vi "open_pneumatics.vi"(8 "error in (no error)":errorcluster) -> (0 "error out":errorcluster)   [LabVIEW 2020]
uses:
  <vilib>/Rock Robotics/WPI/Solenoid/WPI_SolenoidChannel.ctl
  <vilib>/Rock Robotics/WPI/Utilities/WPI_GetSetVariantRefNum.vi
  <vilib>/Rock Robotics/WPI/Solenoid/WPI_SolenoidOpenDouble.vi
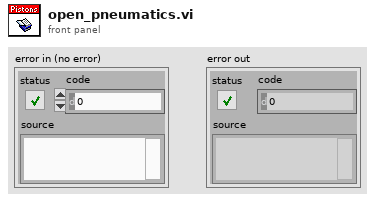
[diagram p1: front panel]
types:
  T1 = typedef "WPI_CompressorDevRef.ctl" = cluster{"DevStatus":errorcluster, "Pneumatics Control Module":u8}
  T2 = typedef "WPI_SolenoidChannel.ctl" = enum8{"Solenoid 0", "Solenoid 1", "Solenoid 2", "Solenoid 3", "Solenoid 4", "Solenoid 5", "Solenoid 6", "Solenoid 7", "Solenoid 8", "Solenoid 9", "Solenoid 10", "Solenoid 11", "Solenoid 12", "Solenoid 13", "Solenoid 14", "Solenoid 15", "Invalid"}
  T3 = typedef "WPI_SolenoidDevRef.ctl" = cluster{"DevStatus":errorcluster, "Pneumatics Control Module":u8, "Forward Solenoid Channel":T2, "Reverse Solenoid Channel":T2}
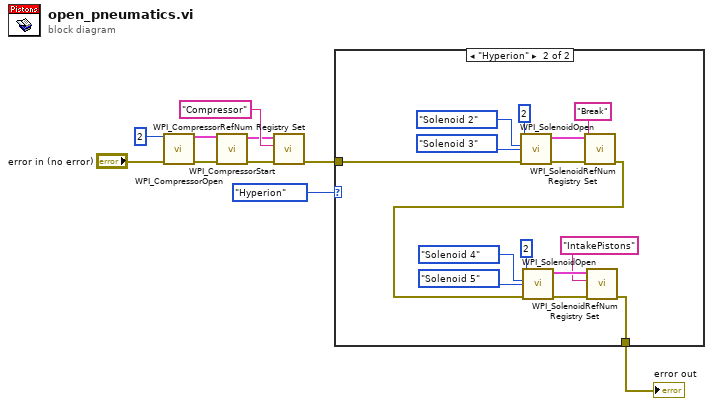
[diagram p0: block diagram]
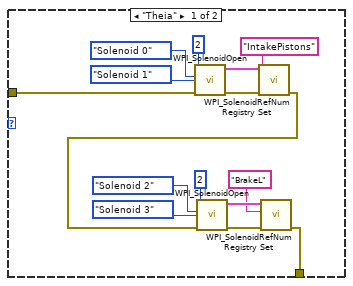
[diagram p2: hidden frame]
diagram:
  n1 = call <vilib>:"WPI_CompressorOpen.vi"("Pneumatics device (def)"=u8 2, "error in (no error)"="error in (no error)") -> ("CompressorDevRef"=w5:T1, "error out"=w6:errorcluster)  [unwired: 12 in]
  n2 = call <vilib>:"WPI_CompressorStart.vi"("error in (no error)"=w6, "CompressorDevRef"=w5) -> ("error out"=w3:errorcluster, "CompressorDevRef"=w4:T1)  [unwired: 8 in]
  n3 = call <vilib>:"WPI_CompressorRefNum Registry Set.vi"("error in (no error)"=w3, "refnum name"="Compressor", "CompressorDevRef"=w4) -> ("error out"=w10:errorcluster)  [unwired: 7 in, 1 out]
  n4 = case shown="\"Hyperion\"" enum16{"Theia", "Hyperion"}."Hyperion" {
    tunnel: w10 -> [w25 w40]
    tunnel: [w11 w26] -> w2
    frame "Theia" {
      n5 = call-poly <vilib>:"WPI_SolenoidOpen.vi"("error in (no error)"=w25, "Reverse Solenoid Channel"=WPI_SolenoidChannel."Solenoid 1", "Forward Solenoid Channel"=WPI_SolenoidChannel."Solenoid 0", "Pneumatics Device (def)"=u8 2) -> ("error out"=w12:errorcluster, "SolenoidDevRef"=w13:T3)  [unwired: 6 in]
      n6 = call <vilib>:"WPI_SolenoidRefNum Registry Set.vi"("error in (no error)"=w12, "refnum name"="IntakePistons", "SolenoidDevRef"=w13) -> ("error out"=w24:errorcluster)  [unwired: 7 in, 1 out]
      n7 = call-poly <vilib>:"WPI_SolenoidOpen.vi"("error in (no error)"=w24, "Reverse Solenoid Channel"=WPI_SolenoidChannel."Solenoid 3", "Forward Solenoid Channel"=WPI_SolenoidChannel."Solenoid 2", "Pneumatics Device (def)"=u8 2) -> ("error out"=w23:errorcluster, "SolenoidDevRef"=w22:T3)  [unwired: 6 in]
      n8 = call <vilib>:"WPI_SolenoidRefNum Registry Set.vi"("error in (no error)"=w23, "refnum name"="BrakeL", "SolenoidDevRef"=w22) -> ("error out"=w11:errorcluster)  [unwired: 7 in, 1 out]
    }
    frame "Hyperion" {
      n9 = call-poly <vilib>:"WPI_SolenoidOpen.vi"("error in (no error)"=w40, "Reverse Solenoid Channel"=WPI_SolenoidChannel."Solenoid 3", "Forward Solenoid Channel"=WPI_SolenoidChannel."Solenoid 2", "Pneumatics Device (def)"=u8 2) -> ("error out"=w27:errorcluster, "SolenoidDevRef"=w28:T3)  [unwired: 6 in]
      n10 = call <vilib>:"WPI_SolenoidRefNum Registry Set.vi"("error in (no error)"=w27, "refnum name"="Break", "SolenoidDevRef"=w28) -> ("error out"=w39:errorcluster)  [unwired: 7 in, 1 out]
      n11 = call-poly <vilib>:"WPI_SolenoidOpen.vi"("error in (no error)"=w39, "Reverse Solenoid Channel"=WPI_SolenoidChannel."Solenoid 5", "Forward Solenoid Channel"=WPI_SolenoidChannel."Solenoid 4", "Pneumatics Device (def)"=u8 2) -> ("error out"=w38:errorcluster, "SolenoidDevRef"=w37:T3)  [unwired: 6 in]
      n12 = call <vilib>:"WPI_SolenoidRefNum Registry Set.vi"("error in (no error)"=w38, "refnum name"="IntakePistons", "SolenoidDevRef"=w37) -> ("error out"=w26:errorcluster)  [unwired: 7 in, 1 out]
    }
  }
  "error out" <- w2
